vi "SubSystems.vi"(8 "error in":errorcluster) -> ()   [LabVIEW 2019]
doc: "This VI calls the various robot subsystems that will then run in parallel. New subSystems will automatlically script code to make the call."
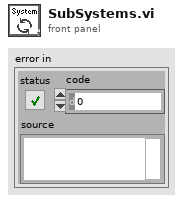
[diagram p1: front panel]
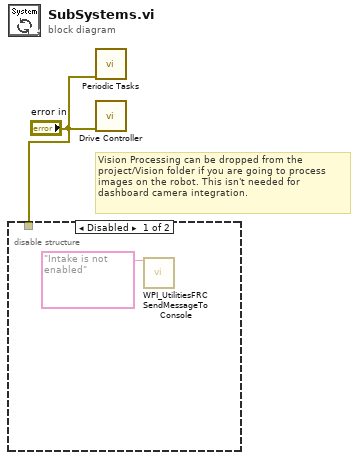
[diagram p0: block diagram]
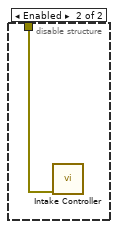
[diagram p2: hidden frame]
diagram:
  # "Vision Processing can be dropped from the\nproject/Vision folder if you are going to process\nimages on the robot. This isn't needed for\ndashboard camera integration."
  n1 = disable-structure shown="Disabled" {
    disable-tunnel: "error in" -> [_ w3]
    frame Disabled {
      n2 = call <vilib>:"WPI_UtilitiesFRC SendMessageToConsole.vi"("Message"="Intake is not enabled") -> ()  [unwired: 14 in, 1 out]
    }
    frame Enabled {
      n3 = call "Intake Controller.vi"("error in"=w3) -> ()  [unwired: 11 in]
    }
  }
  n4 = call "Periodic Tasks.vi"("error in"="error in") -> ()  [unwired: 1 in, 10 out]
  n5 = call "Drive Controller.vi"("error in"="error in") -> ()  [unwired: 11 in]
